vi "Engine - Generic - Medium Pressure Common Rail Host.vi"() -> ()   [LabVIEW 2015, in "ECS-Host.lvlib"]
uses:
  ECS-Host.lvlib
  <vilib>/addons/Software Calibration Management/XControls/TBL1D.xctl
  <vilib>/addons/Software Calibration Management/XControls/SubHost.xctl
  <vilib>/addons/Software Calibration Management/XControls/TBL2D.xctl
panel:
  out "FQVDurAngle_PIDActive":bool
  out "FQVDur_Des":sgl caption="[]" format="%#.2f"
  in  "FQVWindowEnd":sgl caption="[]" format="%#.2f"
  in  "FQVWindowStart":sgl caption="[DBTDC]" format="%#.2f"
  out "CamAdv":sgl caption="[CAD]" format="%#.2f"
  in  "FQVDur_Man":sgl caption="[]" format="%#.2f"
  in  "FQVDur_ManE":bool
  in  "FQVDur_Min":sgl caption="[]" format="%#.2f"
  in  "FQVDur_Max":sgl caption="[]" format="%#.2f"
  in  "FQVCtrl_E":bool
  out "RailP":sgl caption="[bar]" min=0 max=0.2 step=0.001 format="%#.3f"
  out "RailPStp":sgl caption="[bar]" min=0 max=0.2 step=0.001 format="%#.3f"
  in  "_FQV/HPV Tab Control":enum32{"FQV PID", "FQV Feed Forward"}(tab)
  in  "FQVDurAngle_NonPIDFFTbl":cluster{"X":sgl[], "Y":sgl[]}(xcontrol) caption="[CAD]"
  out "FQVDurAngle_PIDOut":sgl caption="[CAD]" max=50
  out "FQVDurAngle_FFTblOut":sgl caption="[CAD]" format="%#.2f"
  in  "FQVDurAngle_Kc":sgl caption="[CAD/bar]" format="%#.3g"
  in  "FQVDurAngle_Ti":sgl caption="[min]" format="%#.3g"
  in  "FQVDurAngle_Td":sgl caption="[min]" format="%#.3g"
  in  "FQVDurAngle_PIDMax":sgl caption="[CAD]" max=50 format="%#.2f"
  in  "FQVDurAngle_PIDMin":sgl caption="[CAD]" format="%#.2f"
  out "FQVDurAngle_KpOut":sgl(slide) caption="FQV_ Kc Action" max=0 scale=0.0..100.0 scale format="%#.2f"
  out "FQVDurAngle_TiOut":sgl(slide) caption="FQV_ Ti Action" max=0 scale=0.0..100.0 scale format="%#.2f"
  out "FQVDurAngle_TdOut":sgl(slide) caption="FQV_ Td Action" max=0 scale=0.0..100.0 scale format="%#.2f"
  in  "FQVDurAngle_FFTbl":cluster{"X":sgl[], "Y":sgl[], "Z":sgl[][]}(xcontrol)
  in  "RPC Plot":T1(xcontrol)
  in  "FQVEndTiming":sgl caption="[DBTDC]" format="%#.2f"
  out "RailP_Fault":bool
  in  "FQVDurAngle_Man":sgl caption="[]" format="%#.2f"
  in  "FQVDurAngle_ManE":bool
  out "FQVDurAngle_Calc":sgl caption="[]" min=0 max=0.2 step=0.001 format="%#.3f"
  out "FQVStartTiming_Des":sgl caption="[]" format="%#.2f"
  in  "FQVDurAngle_Min":sgl caption="[]" format="%#.2f"
  in  "FQVDurAngle_Max":sgl caption="[CAD]" format="%#.2f"
  in  "FQVDurAngle_PIDE":bool
  in  "RailP_MaxThresh":sgl caption="[bar]" min=0 max=0.2 step=0.001 format="%#.3f"
  in  "MPCR_FaultClear":bool
  # "+"
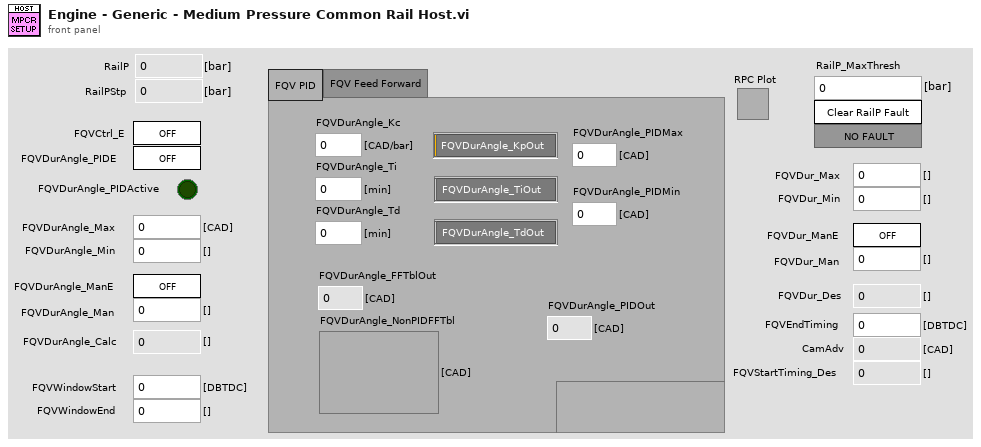
[diagram p1: front panel]
types:
  T1 = cluster{"Name":string, "Host VI":path, "Pairing File":path, "Display Name":string}
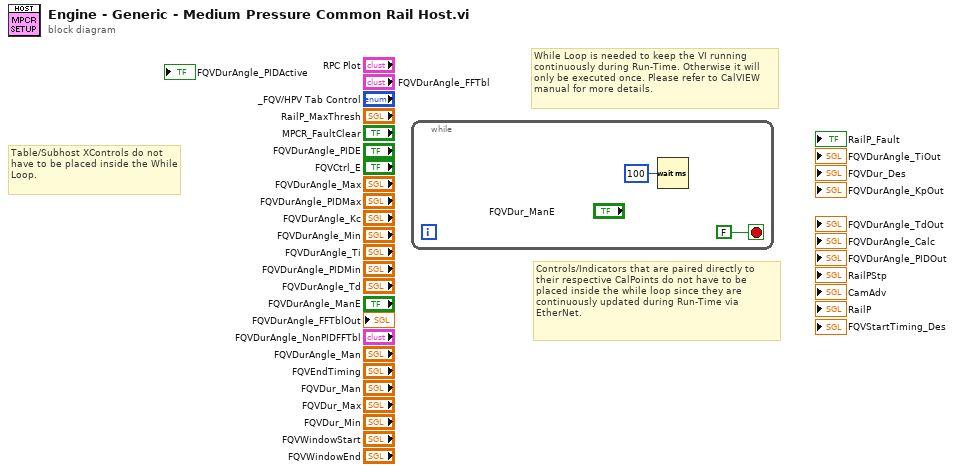
[diagram p0: block diagram]
diagram:
  # "Table/Subhost XControls do not have to be placed inside the While Loop."
  # "While Loop is needed to keep the VI running\ncontinuously during Run-Time. Otherwise it will only be executed once. Please refer to CalVIEW manual for more details."
  # "Controls/Indicators that are paired directly to their respective CalPoints do not have to be placed inside the while loop since they are continuously updated during Run-Time via EtherNet."
  n1 = while {
    stop <- FALSE stop-if-true
    n2 = Wait (ms)(milliseconds to wait=u32 100) -> ()  [unwired: 1 out]
  }
